vi "Get Multi.vi"(0 "Display State In":T1, 5 "Value In":i16, 9 "Container State":T2, 11 "error in (no error)":errorcluster) -> (4 "Display State Out":T1, 6 "Value Out":i16, 8 "mixed":bool, 15 "error out":errorcluster)   [LabVIEW 2015, in "KRing.xctl"]
uses:
  KRing.xctl
  <vilib>/_xctls/Container State.ctl
  State.ctl
  <vilib>/_xctls/XControlSupport.lvlib
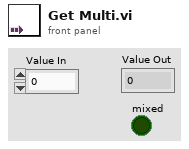
[diagram p1: front panel]
types:
  T1 = typedef "KRing.xctl/State.ctl" = cluster{"mixed":bool, "Value":i16, "Ring":refnum<vi>}
  T2 = typedef "XControlSupport.lvlib/Container State.ctl" = cluster{"Indicator?":bool, "Run Mode?":bool, " Refnum":refnum<vi>}
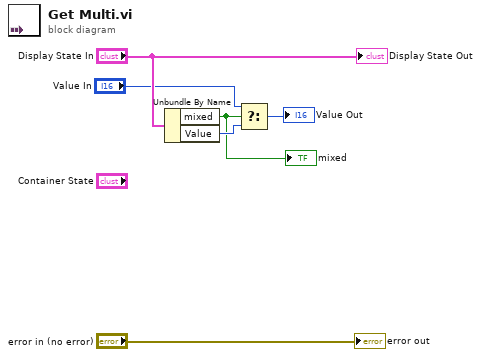
[diagram p0: block diagram]
diagram:
  n1 = Unbundle By Name("Display State In") -> ("mixed"=w1:bool, "Value"=w3:i16)
  "mixed" <- w1
  n2 = Select(t="Value In", s=w1, f=w3) -> (s? t:f=→"Value Out":i16)
  "Display State Out" <- "Display State In"
  "error out" <- "error in (no error)"
